vi "Find Workspace.vi"(8 "error in (no error)":errorcluster, 10 "Control In":T2={"I-O.lvclass"=refnum, "Motion.lvclass"=refnum, "Dispenser.lvclass"=refnum}, 11 "Component.lvclass":refnum<class "8 Inch Component Tray.lvclass">) -> (0 "error out":errorcluster, 1 "Workspace":T1, 2 "Control Out":T2, 3 "Workspace Out":refnum<class "8 Inch Component Tray.lvclass">)   [LabVIEW 2016, in "8 Inch Component Tray.lvclass"]
uses:
  8 Inch Component Tray.lvclass
  Controller/Controllers.ctl
  Controller/I-O/I-O.lvclass
  Controller/Motion/A3200/A3200.lvclass
  Controller/Dispenser/Dispenser.lvclass
  Controller/Motion/Motion.lvclass
  Workspace.ctl
  Component/Component Tray.lvclass
  Controller/Controller.lvclass
  Fixture.lvclass
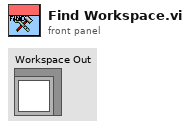
[diagram p1: front panel]
types:
  T1 = typedef "Fixture.lvclass/Workspace.ctl" = cluster{"XYZTheta":dbl[], "Workspace Valve":i32, "Workspace Sensor":i32}
  T2 = typedef "Controller.lvclass/Controllers.ctl" = cluster{"I-O.lvclass":refnum<class "I-O.lvclass">, "Motion.lvclass":refnum<class "Motion.lvclass">, "Dispenser.lvclass":refnum<class "Dispenser.lvclass">}
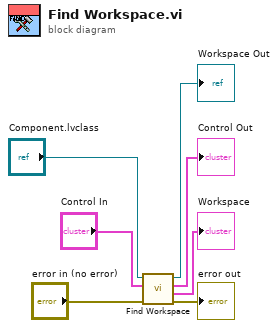
[diagram p0: block diagram]
diagram:
  n1 = call-parent "Find Workspace.vi"("error in (no error)"="error in (no error)", "Control In"="Control In", "Component.lvclass"="Component.lvclass") -> ("error out"=→"error out":errorcluster, "Workspace"=→"Workspace":T1, "Control Out"=→"Control Out":T2, "Workspace Out"=→"Workspace Out":refnum<class "8 Inch Component Tray.lvclass">)  [unwired: 5 in]
